vi "Save_to_Project.vi"(8 "error in (no error)":errorcluster, 9 "index":i32, 10 "buildObject":T1, 11 "AB_Source_Container in":refnum<class "AB_Source_Container.lvclass">) -> (0 "error out":errorcluster, 3 "AB_Source_Container out":refnum<class "AB_Source_Container.lvclass">)   [LabVIEW 2020, in "AB_Source_Container.lvclass"]
uses:
  <vilib>/AppBuilder/AB_Classes/Source/Container/AB_Source_Container.lvclass
  <resource>/Framework/Providers/API/ItemRef.ctl
  <vilib>/AppBuilder/RW_Project/AB_RW_Project_PropBag_Action.ctl
  <vilib>/AppBuilder/RW_Project/AB_RW_Project_Source_Container_Data.ctl
  <vilib>/AppBuilder/AB_Classes/Source/Container/AB_Source_Container.lvclass/AB_Source_Container.ctl
  <vilib>/AppBuilder/AB_Classes/Source/AB_Source.lvclass
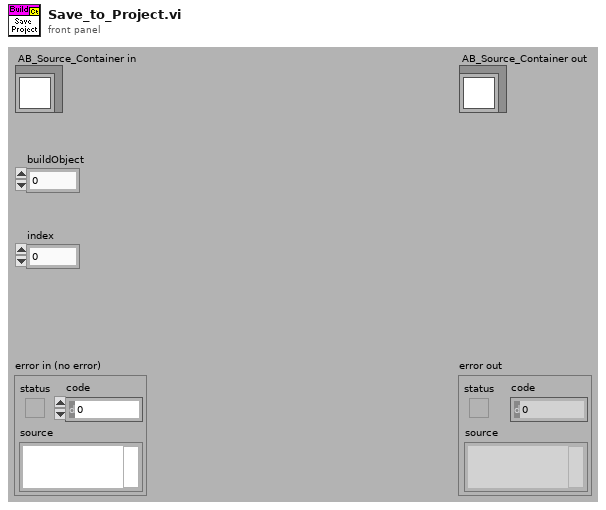
[diagram p1: front panel]
types:
  T1 = typedef "ItemRef.ctl" = u64
  T2 = typedef "AB_RW_Project_PropBag_Action.ctl" = enum16{"read", "write", "clear", "readPrevious", "writePrevious", "clearPrevious"}
  T3 = typedef "AB_RW_Project_Source_Container_Data.ctl" = cluster{"applyInclusion":bool, "applyDestination":bool, "applyProperties":bool, "applyPassword":bool, "applyPrefix":bool, "applySaveSetttings":bool, "dependentDestinationIndex":i32}
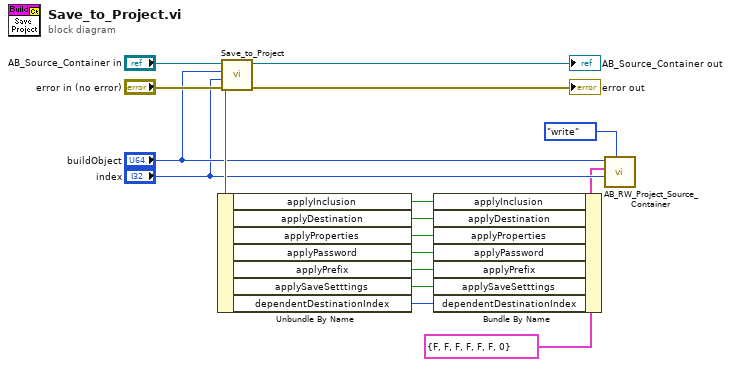
[diagram p0: block diagram]
diagram:
  n1 = call-parent "Save_to_Project.vi"("error in (no error)"="error in (no error)", "index"="index", "buildObject"="buildObject", "AB_Source in"="AB_Source_Container in") -> ("error out"=→"error out":errorcluster, "AB_Source out"=w13:refnum<class "AB_Source_Container.lvclass">)  [unwired: 6 out]
  "AB_Source_Container out" <- w13
  n2 = Unbundle By Name(w13) -> ("applyInclusion"=w9:bool, "applyDestination"=w8:bool, "applyProperties"=w7:bool, "applyPassword"=w6:bool, "applyPrefix"=w3:bool, "applySaveSetttings"=w2:bool, "dependentDestinationIndex"=w1:i32)
  n3 = Bundle By Name(cluster=T3 {"applyInclusion"=FALSE, "applyDestination"=FALSE, "applyProperties"=FALSE, "applyPassword"=FALSE, "applyPrefix"=FALSE, "applySaveSetttings"=FALSE, "dependentDestinationIndex"=0} ("dataSource in"), "applyInclusion"=w9, "applyDestination"=w8, "applyProperties"=w7, "applyPassword"=w6, "applyPrefix"=w3, "applySaveSetttings"=w2, "dependentDestinationIndex"=w1) -> (w5:T3)
  n4 = call <vilib>:"AB_RW_Project_Source_Container.vi"("action"=AB_RW_Project_PropBag_Action."write", "index in"="index", "dataSource in"=w5, "buildObject"="buildObject") -> ()  [unwired: 1 in, 7 out]
